vi "MTM2_putSample_systemStatus.vi"(8 "error in (no error)":errorcluster, 11 "systemStatus_Ctl":T1={"statusBits[72]"=[0, 0, 0, 0, 0, 0, 0, 0, 0, 0, 0, 0, 0, 0, 0, 0, 0, 0, 0, 0, 0, 0, 0, 0, 0, 0, 0, 0, 0, 0, 0, 0, 0, 0, 0, 0, 0, 0, 0, 0, 0, 0, 0, 0, 0, 0, 0, 0, 0, 0, 0, 0, 0, 0, 0, 0, 0, 0, 0, 0, 0, 0, 0, 0, 0, 0, 0, 0, 0, 0, 0, 0]}) -> (0 "error out":errorcluster, 2 "function return":i32, 3 "systemStatus_Ctl out":T1)   [LabVIEW 2018, in "SALLV_MTM2.lvlib"]
doc: "int MTM2_shm_putSample_systemStatusLV(MTM2_systemStatusLV *systemStatus_Ctl );"
uses:
  SALLV_MTM2.lvlib
  DataTypes/systemStatus.ctl
  SALLV_MTM2.so
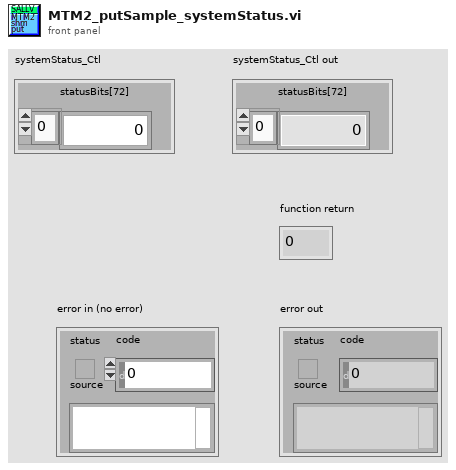
[diagram p1: front panel]
types:
  T1 = typedef "SALLV_MTM2.lvlib/systemStatus.ctl" = cluster{"statusBits[72]":u32[]}
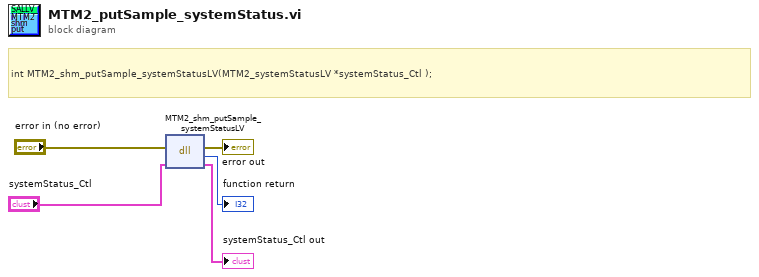
[diagram p0: block diagram]
diagram:
  # "int MTM2_shm_putSample_systemStatusLV(MTM2_systemStatusLV *systemStatus_Ctl );"
  n1 = dll-call lib="home/ttsai/Document/salApiMTM2/SALLV_MTM2/SALLV_MTM2.*" fn="MTM2_shm_putSample_systemStatusLV"(error in="error in (no error)", "systemStatus_Ctl"="systemStatus_Ctl") -> (error out=→"error out":errorcluster, →"function return":i32, "systemStatus_Ctl"=→"systemStatus_Ctl out":T1)  [unwired: 2 in, 1 out]
